vi "ATF Pump Parameter GUI V1.1.vi"() -> ()   [LabVIEW 2022 SP3]
panel:
  in  "Exit":bool
  out "A_NDB":dbl format="%.2f"
  out "A_DB":dbl format="%.2f"
  out "V_NDB":dbl format="%.2f"
  out "V_DB":dbl format="%.2f"
  out "H_NDB":dbl format="%.2f"
  out "H_DB":dbl format="%.2f"
  out "A NDB 2":dbl format="%#.2f"
  out "A DB 2":dbl format="%#.2f"
  out "V_NDB 2":dbl format="%#.2f"
  out "V DB 2":dbl format="%#.2f"
  out "H NDB 2":dbl format="%#.2f"
  out "H DB  2":dbl format="%#.2f"
  out "Speed(RPM)":dbl format="%#.2f"
  out "Torque":dbl format="%#.2f"
  out "PUMP HEAD   =":dbl format="%#.2f"
  out "Speed (RPM)":dbl format="%#.2f"
  out "F_SC_RTD (K)":dbl format="%#.2f"
  out "F-SC-PT(bar)":dbl format="%#.2f"
  out "F_RTD_1013 (K)":dbl format="%#.2f"
  out "F_PT_1013a (bar)":dbl format="%#.2f"
  out "F_RTD_1011 (K)":dbl format="%#.2f"
  out "F_PT_1011a (bar)":dbl format="%#.2f"
  out "F_FM-1010 (g/s)":dbl format="%#.2f"
  out "F_PT_1013b (bar)":dbl format="%#.2f"
  out "F_PT_1011b (bar)":dbl format="%#.2f"
  out "Current (A)":dbl format="%#.2f"
  out "Voltage (V)":dbl format="%#.2f"
  out "D_Dyna_PT (bar)":dbl format="%#.2f"
  out "S_Dyna_PT (bar)":dbl format="%#.2f"
  out "F_PT_9 (bar)":dbl format="%#.2f"
  out "F_PT_8 (bar)":dbl format="%#.2f"
  out "F_PT_5 (bar)":dbl format="%#.2f"
  out "F_PT_6 (bar)":dbl format="%#.2f"
  out "F_PT_7 (bar)":dbl format="%#.2f"
  out "F_PT_4 (bar)":dbl format="%#.2f"
  out "F_PT_1 (bar)":dbl format="%#.2f"
  out "F_PT_2 (bar)":dbl format="%#.2f"
  out "F_PT_3 (bar)":dbl format="%#.2f"
  out "ND B 2 (K)":dbl format="%#.2f"
  out "RTD OUT (K)":dbl format="%#.2f"
  out "ND B 1(K)":dbl format="%#.2f"
  out "DE Bearing T (C))":dbl format="%#.2f"
  out "Motor Outer\n body Temp(C)":dbl format="%#.2f"
  out "NDE Bearing T (C)":dbl format="%#.2f"
  out "P_TC5 (k)":dbl format="%#.2f"
  out "P_TC4 (k)":dbl format="%#.2f"
  out "P_TC3 (K)":dbl format="%#.2f"
  out "P_RTD (k)":dbl format="%#.2f"
  out "P_TC2 (k)":dbl format="%#.2f"
  out "P_TC1 (k)":dbl format="%#.2f"
  # "ATF RIG PARAMETERS"
  # "THERMAL DATA"
  # "PRESSURE DATA"
  # "CRITICAL DATA"
  # "VIBRATION DATA"
  # "MOTOR"
  # "NDB"
  # "DB"
  # "g"
  # "g"
  # "H"
  # "g"
  # "V"
  # "g"
  # "g"
  # "g"
  # "A"
  # "PUMP"
  # "BEARING"
  # "PUMP"
  # "g"
  # "H"
  # "g"
  # "g"
  # "V"
  # "g"
  # "g"
  # "A"
  # "g"
  # "TORQUE METER"
  # "DRIVE PARAMETERS"
  # "F_S_Uol_PT"
  # "F_S_Dol_PT"
  # "F_SC_PT"
  # "F_SF_PT"
  # "F_V_PT1"
  # "F_V_PT2"
  # "F_V_PT3"
  # "F_V_PT4"
  # "F_D_PT"
  # "MOTOR"
  # "PUMP"
  # "Version:V0.1"
  # "Release Date:17/10/2024"
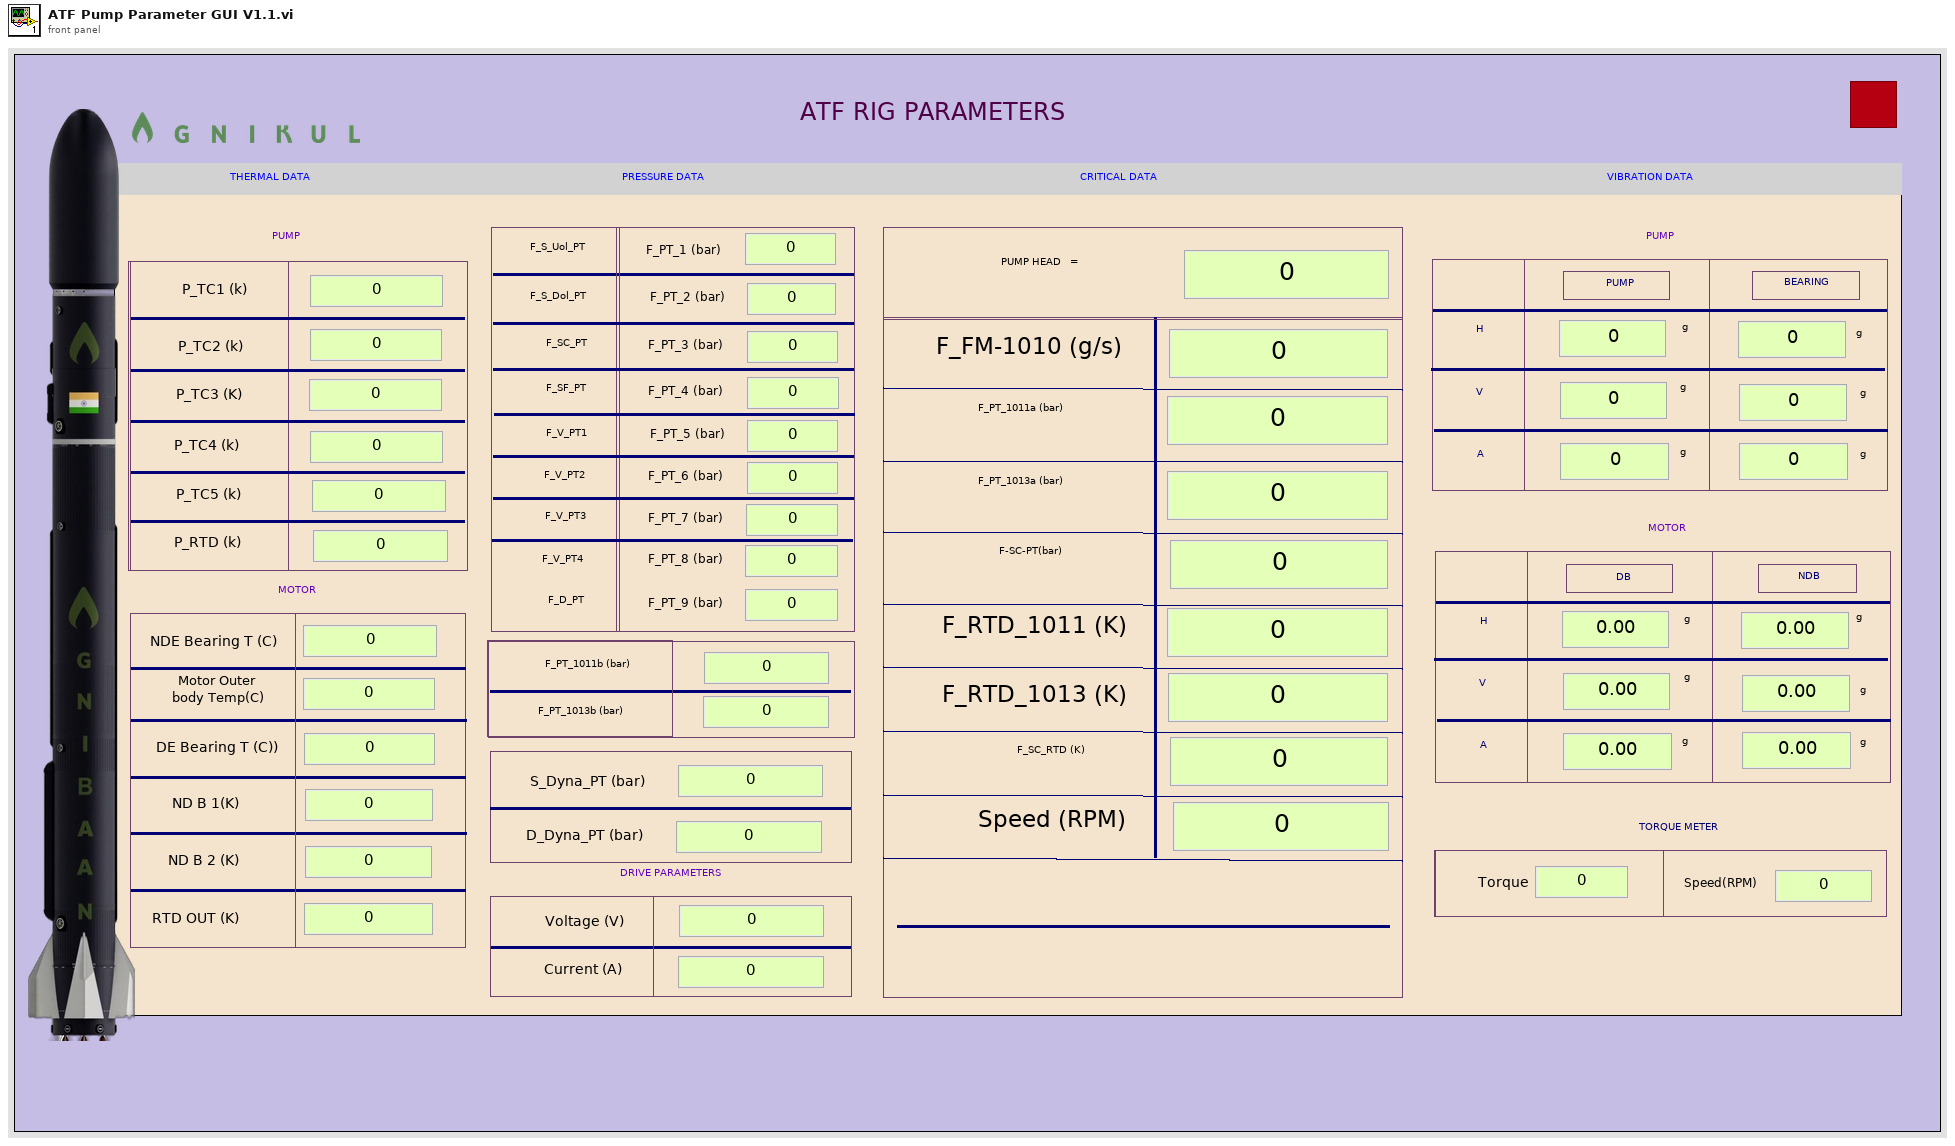
[diagram p1: front panel]
types:
  T1 = typedef "SeCrTS-Notifier Ref.ctl" = cluster{"Pump":refnum<notifier>, "Storage":refnum<notifier>}
  T2 = cluster{"AI_V_Data":waveform(dbl)[][], "AI_C_Data":waveform(dbl)[][], "AO_Data":waveform(dbl)[][], "DO_Data":waveform(dbl)[][], "DI_Data":digitalwaveform[][], "ACC_Data":waveform(dbl)[][], "TC Data":waveform(dbl)[][], "Drive_A_C":waveform(dbl)[][], "Drive_A_D":waveform(dbl)[][], "AI_V Rms":waveform(dbl)[][]}
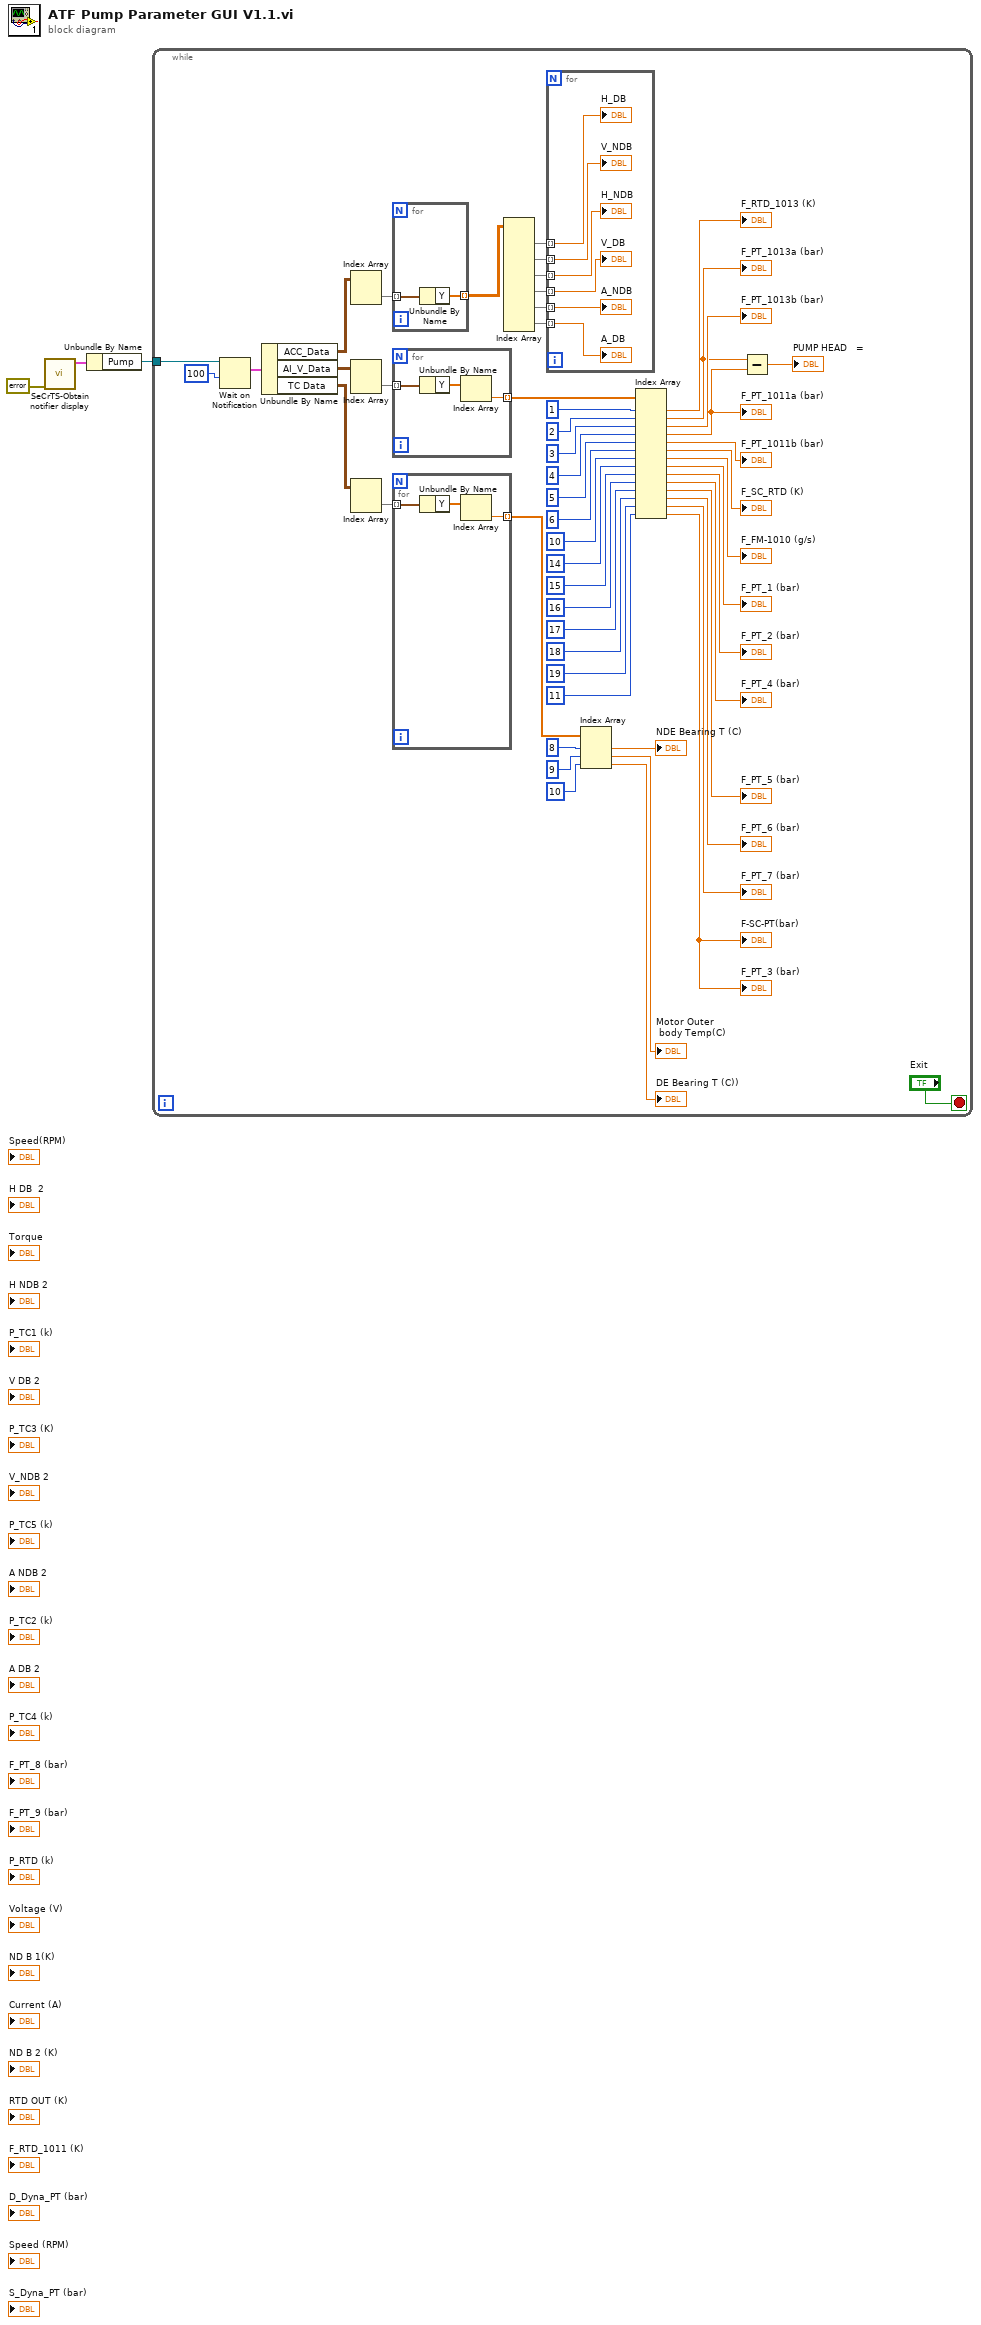
[diagram p0: block diagram]
diagram:
  n1 = call "SeCrTS-Obtain notifier display.vi"("error in (no error)"=errorcluster {"status"=FALSE, "code"=0, "source"=""}) -> ("NOT DIS Out"=w3:T1)  [unwired: 9 in, 1 out]
  n2 = Unbundle By Name(w3) -> ("Pump"=w2:refnum<notifier>)
  n3 = while {
    tunnel: w2 -> [w13]
    stop <- "Exit" stop-if-true
    n4 = Wait on Notification(notifier=w13, timeout in ms (-1)=100) -> (notification=w12:T2)  [unwired: 2 in, 3 out]
    n5 = Unbundle By Name(w12) -> ("ACC_Data"=w11:waveform(dbl)[][], "AI_V_Data"=w9:waveform(dbl)[][], "TC Data"=w7:waveform(dbl)[][])
    n6 = Index Array(array=w11) -> (element=w10:waveform(dbl)[])  [unwired: 2 in]
    n7 = Index Array(array=w9) -> (element=w8:waveform(dbl)[])  [unwired: 2 in]
    n8 = Index Array(array=w7) -> (element=w6:waveform(dbl)[])  [unwired: 2 in]
    n9 = for {
      tunnel: w10 -> [w67] mode=indexing
      tunnel: [w68] -> w42 mode=indexing
      n10 = Unbundle By Name(w67) -> ("Y"=w68:dbl[])
    }
    n11 = for {
      tunnel: w8 -> [w70] mode=indexing
      tunnel: [w69] -> w50 mode=indexing
      n12 = Unbundle By Name(w70) -> ("Y"=w71:dbl[])
      n13 = Index Array(array=w71) -> (element=w69:dbl)  [unwired: 1 in]
    }
    n14 = for {
      tunnel: [w66] -> w20 mode=indexing
      tunnel: w6 -> [w65] mode=indexing
      n15 = Unbundle By Name(w65) -> ("Y"=w64:dbl[])
      n16 = Index Array(array=w64) -> (element=w66:dbl)  [unwired: 1 in]
    }
    n17 = Index Array(array=w42) -> (element #1=w41:dbl[], element #2=w40:dbl[], element #3=w39:dbl[], element #4=w38:dbl[], element #5=w37:dbl[], element #6=w36:dbl[])  [unwired: 12 in]
    n18 = for {
      tunnel: w41 -> [w63] mode=indexing
      tunnel: w40 -> [w62] mode=indexing
      tunnel: w39 -> [w61] mode=indexing
      tunnel: w38 -> [w60] mode=indexing
      tunnel: w37 -> [w59] mode=indexing
      tunnel: w36 -> [w58] mode=indexing
      "H_DB" <- w63
      "H_NDB" <- w61
      "V_DB" <- w60
      "V_NDB" <- w62
      "A_DB" <- w58
      "A_NDB" <- w59
    }
    n19 = Index Array(array=w20, index #1=8 ("index"), index #2=9 ("index"), index #3=10 ("index")) -> (element #1=→"NDE Bearing T (C)":dbl, element #2=→"Motor Outer\n body Temp(C)":dbl, element #3=→"DE Bearing T (C))":dbl)
    n20 = Index Array(array=w50, index #1=1 ("index"), index #2=2 ("index"), index #3=3 ("index"), index #4=4 ("index"), index #5=5 ("index"), index #6=6 ("index"), index #7=10 ("index"), index #8=14 ("index"), index #9=15 ("index"), index #10=16 ("index"), index #11=17 ("index"), index #12=18 ("index"), index #13=19 ("index"), index #14=11 ("index")) -> (element #1=→"F_RTD_1013 (K)":dbl, element #2=w44:dbl, element #3=→"F_PT_1013b (bar)":dbl, element #4=w43:dbl, element #5=→"F_PT_1011b (bar)":dbl, element #6=→"F_SC_RTD (K)":dbl, element #7=→"F_FM-1010 (g/s)":dbl, element #8=→"F_PT_1 (bar)":dbl, element #9=→"F_PT_2 (bar)":dbl, element #10=→"F_PT_4 (bar)":dbl, element #11=→"F_PT_5 (bar)":dbl, element #12=→"F_PT_6 (bar)":dbl, element #13=→"F_PT_7 (bar)":dbl, element #14=→"F_PT_3 (bar)" →"F-SC-PT(bar)":dbl)
    "F_PT_1013a (bar)" <- w44
    "F_PT_1011a (bar)" <- w43
    n21 = Subtract(x=w44, y=w43) -> (x-y=→"PUMP HEAD   =":dbl)
  }
